vi "ELM.vi"(0 "VISA resource name":refnum<visa-resource-name>="COM1", 1 "baud rate":u32=9600, 2 "data bits":u16=8 min=5 max=8 step=1, 3 "parity":u16(ring) items=["None", "Odd", "Even", "Mark", "Space"], 4 "stop bits":u16(ring)=10 items=["1.0"=10, "1.5"=15, "2.0"=20], 5 "write":bool, 6 "read":bool=TRUE, 7 "flow control":u16(ring) items=["None"=0, "XON/XOFF"=1, "RTS/CTS"=2, "DTR/DSR"=4], 8 "string to write":string="*IDN?\n") -> (9 "read string":string, 10 "bytes read":u32)   [LabVIEW 2012]
doc: "The Basic Serial Read and Write example performs a Serial Port Read, a Serial Port Write, or a combination of these actions. The user selects the actions (read or write) on the front panel. If both are selected, the VI will write the data first, read data, and then close the VISA session that is opened to the port. This VI will wait until the specified number of bytes is received at the port or until a termination character is read.\n\nINSTRUCTIONS:\n1) Select the serial resource and configuration parameters (baud rate, data bits, parity, stop bits, flow control).\n2) Select the operations to be performed. \n3) Connect the serial port to your device. If no device is available, perform a loopback test by doing one of the following. Short pins 2 and 3 on a RS-232 cable or short pin 4 to pin 8 and pin 5 to pin 9 on a RS-485/422 cable. \n4) Run the VI to see the data read. (The \"read string\" will match the \"string to write\" if a loopback test was performed.)\n\nNote: The parameters set for the serial port must match the parameters of the connected instrument or device. In this example, the bytes to read parameter specifies the number of bytes that the serial port reads. If there were more bytes at the port than the number specified in bytes to read, those bytes would not be read. Also, if you specify to read more bytes than the number of bytes actually read, you might receive a timeout error message.\n\nOn the block diagram, the Configure Serial Port VI sets the configuration parameters. The front panel displays the controls used to configure the basic parameters, such as baud rate, data bits, and parity. Constants configure the other parameters the user probably does not need set. After the VISA Configure Serial Port VI opens the VISA session and configures the port, the VI passes the VISA resource name to other VIs that perform operations on that VISA resource. The VISA Write function sends a command to the serial device and the VISA Read function returns data based on the command. The VISA Close function then closes the reference to the serial device. It is important to close the reference; otherwise communication through with that port through protocols other than VISA might not be possible."
uses:
  <vilib>/Platform/TimedLoop/XDataNode/timing_clust.ctl
  <vilib>/Platform/TimedLoop/XDataNode/nitl_modes.ctl
  <vilib>/Platform/TimedLoop/XDataNode/wakeup.ctl
  <vilib>/Instr/_visa.llb/VISA Configure Serial Port (Instr).vi
  <vilib>/platform/TimedLoop/XDataNode/XDataNode.xnode
  <vilib>/Platform/TimedLoop/XDataNode/XDNodeRunTimeDep.lvlib
panel:
  in  "stop":bool
  in  "delay before read (ms)":u32=500
  # "On Windows/Linux, consider using the Instrument Driver Finder (Help>>Find Instrument Drivers) to search for an instrument driver for your instrument."
  # "Select the serial resource and the operations (Read, Write, or both) to be performed.  If both are selected, the VI will write the data first, read data and then close the VISA session that is opened to the port.  This VI will wait until the specified number of bytes is received at the port or until a termination character is read."
  # "For additional information select File >> VI Properties >> Documentation"
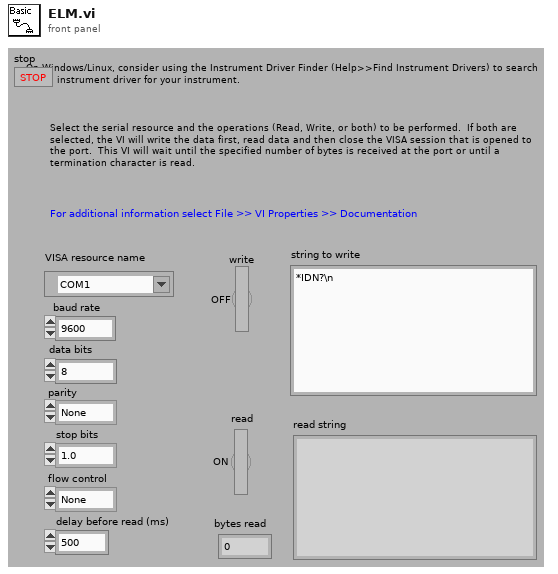
[diagram p1: front panel]
types:
  T1 = typedef "XDNodeRunTimeDep.lvlib/timing_clust.ctl" = cluster{"Expected End [f-1]":u64, "Actual End [f-1]":u64, "Finished Late? [f-1]":bool, "Expected End [i-1]":u64, "Actual End [i-1]":u64, "Finished Late? [i-1]":bool, "Expected Start [i]":u64, "Actual Start [i]":u64, "Expected Start [f]":u64, "Actual Start [f]":u64, "Source Name":string, "Structure Name":string, "Period":i64, "Deadline":i64, "Offset":i64, "Start":i64, "Priority":i32, "Timeout":i32, "Mode":T2, "Wakeup Reason":T3, "Error":errorcluster, "Source Type":string, "Secondary Source Type":string, "Global End Time":u64, "Global Start Time":u64, "Frame Duration":u64, "Iteration Duration":u64, "Assigned CPU":i32, "I/O Scan Engine Mode":u32}
  T2 = typedef "XDNodeRunTimeDep.lvlib/nitl_modes.ctl" = enum32{"No Change", "Process missed periods, maintain original phase", "Discard missed periods, maintain original phase", "Process missed periods, ignore original phase", "Discard missed periods, ignore original phase"}
  T3 = typedef "XDNodeRunTimeDep.lvlib/wakeup.ctl" = enum32{"Normal", "Aborted", "Asynchronous wakeup", "Timing source error", "Timed loop error", "Timeout"}
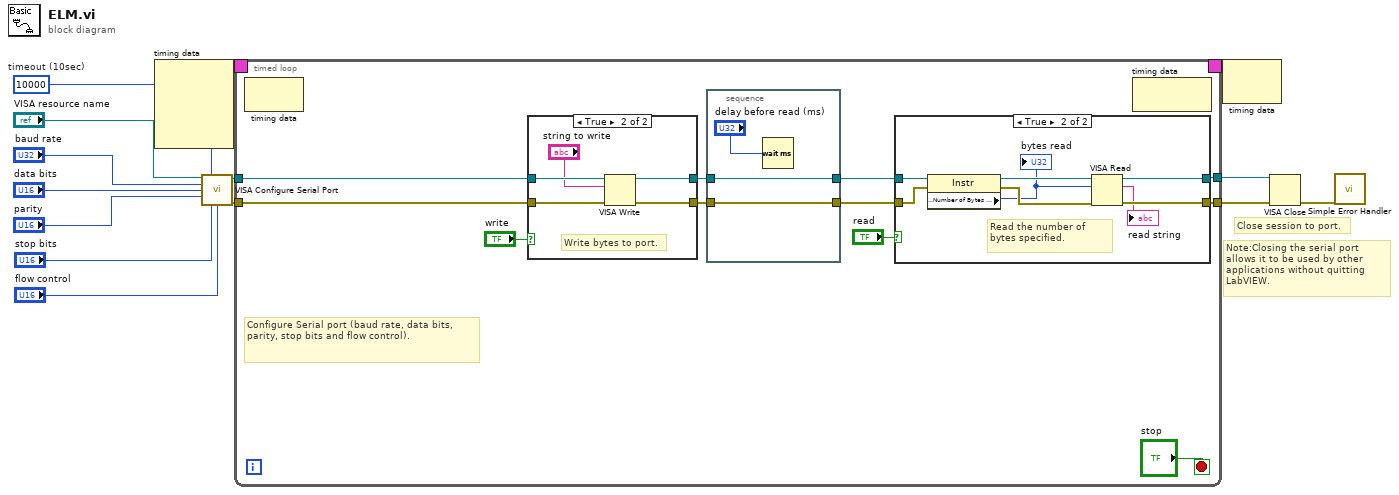
[diagram p0: block diagram]
diagram:
  w6 = u32 10000  # timeout (10sec)
  # "Note:Closing the serial port allows it to be used by other applications without quitting LabVIEW."
  # "Close session to port."
  n1 = node-c288() -> (w2:T1)  [unwired: 4 in]
  n2 = call-poly "VISA Configure Serial Port"("VISA resource name"="VISA resource name", "timeout (10sec)"=w6, "baud rate (9600)"="baud rate", "data bits (8)"="data bits", "parity (0:none)"="parity", "stop bits (10: 1 bit)"="stop bits", "flow control (0:none)"="flow control") -> ("VISA resource name out"=w11:refnum<visa-resource-name>, "error out"=w12:errorcluster)  [unwired: 2 in, 5 out]
  n3 = timed-loop {
    timing: w2 -> [_]
    timing-out: [_] -> w1
    tunnel: w12 -> [w25]
    tunnel: w11 -> [w24]
    tunnel: [w23] -> w10
    tunnel: [w22] -> w9
    stop <- "stop" stop-if-true
    # "Configure Serial port (baud rate, data bits, parity, stop bits and flow control)."
    n4 = node-c288() -> ()  [unwired: 1 in, 1 out]
    n5 = case shown="True" "write" {
      tunnel: [w40 w45] -> w20
      tunnel: w24 -> [w39 w44]
      tunnel: w25 -> [w40 w43]
      tunnel: [w39 w42] -> w18
      frame False {
      }
      frame True {
        # "Write bytes to port."
        n6 = VISA Write(VISA resource name=w44, write buffer="string to write", error in (no error)=w43) -> (VISA resource name out=w42:refnum<visa-resource-name>, error out=w45:errorcluster)  [unwired: 1 out]
      }
    }
    n7 = stacked-sequence {
      tunnel: w20 -> [w38]
      tunnel: [w38] -> w19
      tunnel: w18 -> [w37]
      tunnel: [w37] -> w17
      frame #0 {
        n8 = Wait (ms)(milliseconds to wait="delay before read (ms)") -> ()  [unwired: 1 out]
      }
    }
    n9 = case shown="True" "read" {
      tunnel: w19 -> [w27 w31]
      tunnel: [w27 w35] -> w23
      tunnel: [w26 w34] -> w22
      tunnel: w17 -> [w26 w33]
      frame False {
      }
      frame True {
        # "Read the number of bytes specified."
        n10 = property class="Instr"(reference=w33, error in=w31) -> (reference out=w32:refnum<visa-resource-name>, error out=w30:errorcluster, "Serial Settings:Number of Bytes at Serial Port"=w28:u32)
        "bytes read" <- w28
        n11 = VISA Read(VISA resource name=w32, byte count=w28, error in (no error)=w30) -> (VISA resource name out=w34:refnum<visa-resource-name>, read buffer=→"read string":string, error out=w35:errorcluster)  [unwired: 1 out]
      }
    }
    n12 = node-c288() -> ()  [unwired: 1 in, 1 out]
  }
  n13 = node-c288(w1) -> ()  [unwired: 1 out]
  n14 = VISA Close(VISA resource name=w9, error in (no error)=w10) -> (error out=w8:errorcluster)
  n15 = call <vilib>:"Simple Error Handler.vi"("error in (no error)"=w8) -> ()  [unwired: 1 in, 8 out]
